vi "COM_Data Preprocessing.vi"(7 "Parameters":T1, 8 "error in":errorcluster, 11 "Waveforms IN":waveform(dbl)[](array[waveform])) -> (0 "error out":errorcluster, 3 "Waveforms OUT":waveform(dbl)[](array[waveform]))   [LabVIEW 2017, in "AppPlugins.lvlib" / "EraPlugin.lvclass"]
uses:
  EraPlugin.lvclass
  COM_Preproc Parameters.ctl
  <vilib>/Analysis/2dsp.llb/Decimate (single shot, DBL).vi
  <vilib>/addons/Time Series Analysis/Series Preprocess.llb/TSA Detrend (Waveform).vi
  <vilib>/Analysis/NI_AALPro.lvlib
  <vilib>/addons/System Identification/NI_SysID.lvlib
  <vilib>/addons/_Advanced Signal Processing/NI_AdvSigProcTSA.lvlib
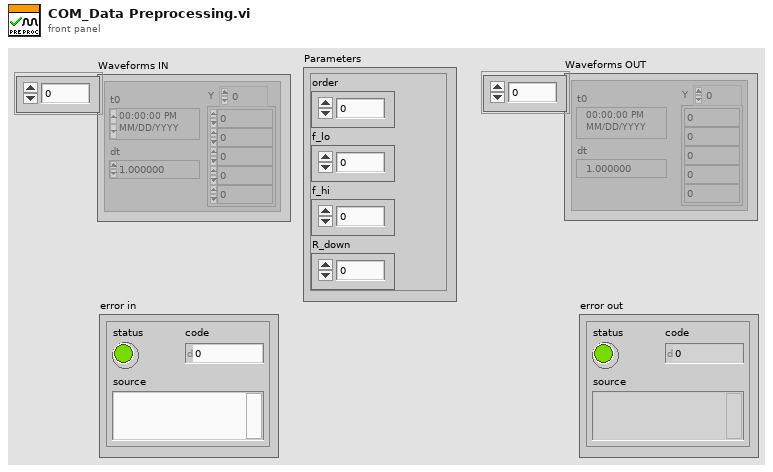
[diagram p1: front panel]
types:
  T1 = typedef "AppPlugins.lvlib/EraPlugin.lvclass/COM_Preproc Parameters.ctl" = cluster{"order":i32, "f_lo":dbl, "f_hi":dbl, "R_down":i32}
  T2 = enum32{"Lowpass", "Highpass", "Bandpass", "Bandstop"}
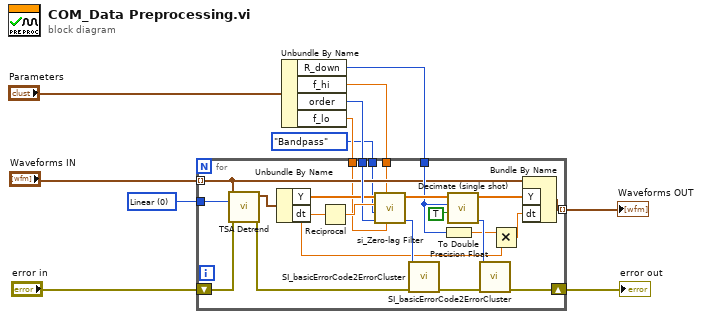
[diagram p0: block diagram]
diagram:
  w3 = u16 0 items=["Linear", "Quadratic", "Cubic", "N-polynomial", "Exponential"] ("method")
  n1 = Unbundle By Name("Parameters") -> ("R_down"=w8:i32, "f_hi"=w7:dbl, "order"=w6:i32, "f_lo"=w2:dbl)
  n2 = for {
    tunnel: w6 -> [w26]
    tunnel: w7 -> [w14]
    tunnel: w8 -> [w25]
    tunnel: "Waveforms IN" -> [w18] mode=indexing
    shift-right: [w24] -> w4
    shift-left: "error in" -> [w19]
    tunnel: [w23] -> w10 mode=indexing
    tunnel: w3 -> [w15]
    tunnel: w2 -> [w13]
    tunnel: T2."Bandpass" ("filter type") -> [w12]
    n3 = call-poly <vilib>:"TSA Detrend.vi"("error in (no error)"=w19, "method"=w15, "Xt"=w18) -> ("error out"=w20:errorcluster, "Xt detrended"=w17:waveform(dbl))  [unwired: 6 in, 1 out]
    n4 = Unbundle By Name(w17) -> ("Y"=w16:dbl[], "dt"=w21:dbl)
    n5 = Reciprocal(x=w21) -> (1/x=w27:dbl)
    n6 = call <vilib>:"si_Zero-lag Filter.vi"("fl"=w13, "fh"=w14, "order"=w26, "filter type"=w12, "sample rate"=w27, "signal in"=w16) -> ("error"=w33:i32, "signal out"=w32:dbl[])  [unwired: 4 out]
    n7 = call <vilib>:"SI_basicErrorCode2ErrorCluster.vi"("error in (no error)"=w20, "error code"=w33) -> ("error out"=w30:errorcluster)  [unwired: 2 in, 7 out]
    n8 = To Double Precision Float(number=w25) -> (double precision float=w28:dbl)
    n9 = call-poly <vilib>:"Decimate (single shot).vi"("averaging"=TRUE, "decimating factor"=w25, "X"=w32) -> ("error"=w31:i32, "Decimated Array"=w29:dbl[])  [unwired: 7 in]
    n10 = call <vilib>:"SI_basicErrorCode2ErrorCluster.vi"("error in (no error)"=w30, "error code"=w31) -> ("error out"=w24:errorcluster)  [unwired: 2 in, 7 out]
    n11 = Multiply(x=w28, y=w21) -> (x*y=w22:dbl)
    n12 = Bundle By Name(cluster=w18, "Y"=w29, "dt"=w22) -> (w23:waveform(dbl))
  }
  "Waveforms OUT" <- w10
  "error out" <- w4
